vi "moveFilterWheel.vi"(6 "Delay between send and receive [ms]":i32=100, 8 "error in (no error)":errorcluster, 9 "position":i32, 10 "locationId":i32, 11 "Monochromator in":refnum<class "Monochromator.lvclass">) -> (0 "error out":errorcluster, 1 "ID":i32, 2 "results-JSON string":string, 3 "Monochromator out":refnum<class "Monochromator.lvclass">)   [LabVIEW 2023, in "Monochromator.lvclass"]
doc: "Move the filter wheel to a position.\n\nlocationId Integer. Specifies which filter wheel to move.\n0 = Filter wheel 1 (Internal)\n1 = Filter wheel 2 (External)\nposition Integer. Position to move the filter wheel."
uses:
  Monochromator.lvclass
  29a0d797-fd6c-43e0-b242-80b21aa51c30.vi
  7fe8abea-6ecd-46de-aa11-ce8637911b6a.vi
  35d46a5a-fd7c-4445-96f4-e877dae8f93b.vi
  <vilib>/JDP Science/JSONtext/Variant to JSON Text.vi
  <vilib>/JDP Science/JSONtext/Set Item.vi
  <vilib>/JDP Science/JSONtext/LVClass Serializer/JSONtext LVClass Serializer.lvclass
  Monochromator.lvclass/Monochromator.ctl
  GenericDevice/GenericDevice.lvclass
panel:
  # "Connector Pane"
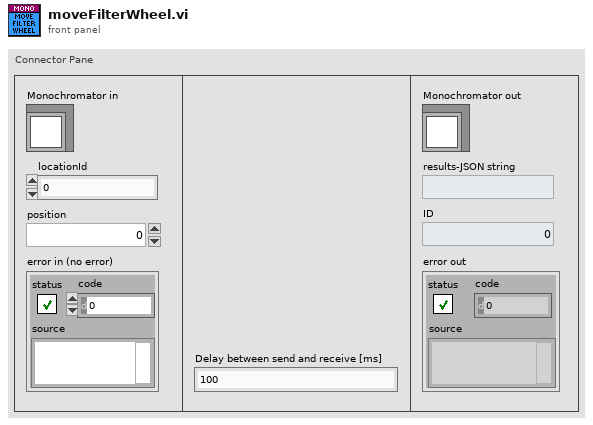
[diagram p1: front panel]
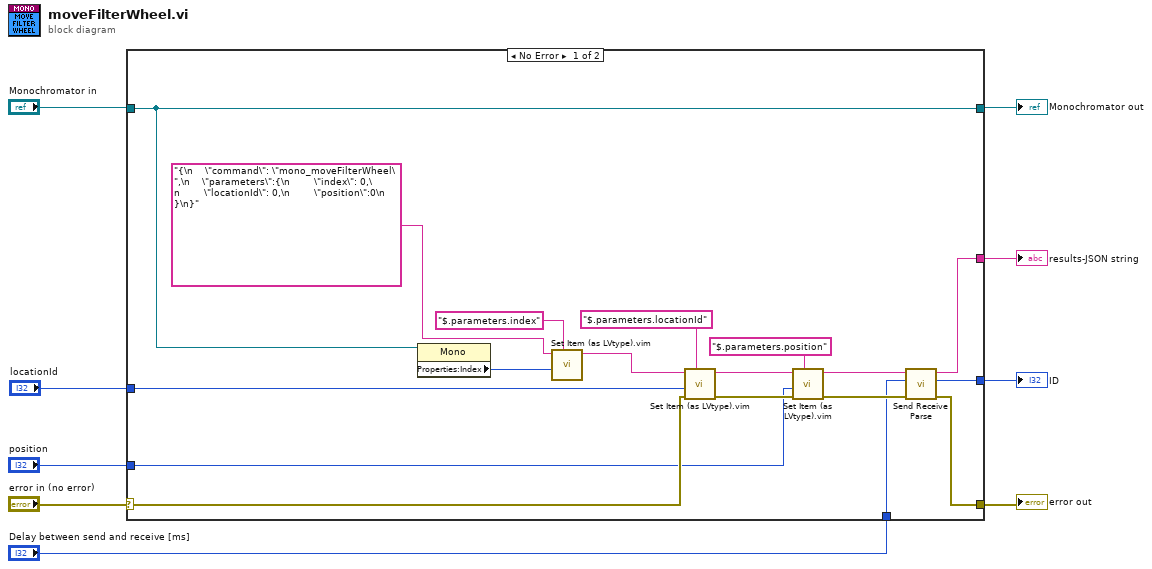
[diagram p0: block diagram]
diagram:
  n1 = case shown="No Error" "error in (no error)" {
    selector: "error in (no error)" -> [w26 w29]
    tunnel: [w23 w29] -> w6
    tunnel: [w15 w28] -> w8
    tunnel: "Monochromator in" -> [w15 w28]
    tunnel: [w25 _] -> w4
    tunnel: [w24 _] -> w5
    tunnel: "position" -> [w17 _]
    tunnel: "Delay between send and receive [ms]" -> [w16 _]
    tunnel: "locationId" -> [w10 _]
    frame No Error {
      n2 = property class="Mono"(reference=w15) -> ("Properties:Index"=w14:i32)  [unwired: 1 in, 2 out]
      n3 = call "Set Item (as LVtype).vim"("$Path or Item Name"="$.parameters.index", "Anything"=w14, "JSON"="{\n    \"command\": \"mono_moveFilterWheel\",\n    \"parameters\":{\n        \"index\": 0,\n        \"locationId\": 0,\n        \"position\":0\n    }\n}") -> ("<JSON>"=w12:string)  [unwired: 5 in, 2 out]
      n4 = call "Set Item (as LVtype).vim"("$Path or Item Name"="$.parameters.locationId", "error in (no error)"=w26, "Anything"=w10, "JSON"=w12) -> ("error out"=w21:errorcluster, "<JSON>"=w19:string)  [unwired: 4 in, 1 out]
      n5 = call "Set Item (as LVtype).vim"("$Path or Item Name"="$.parameters.position", "error in (no error)"=w21, "Anything"=w17, "JSON"=w19) -> ("error out"=w20:errorcluster, "<JSON>"=w18:string)  [unwired: 4 in, 1 out]
      n6 = call "Send Receive Parse.vi"("error in"=w20, "Delay between send and receive [ms]"=w16, "<JSON>"=w18) -> ("error out"=w23:errorcluster, "ID"=w24:i32, "results-JSON string"=w25:string)  [unwired: 6 in]
    }
    frame Error {
    }
  }
  "error out" <- w6
  "Monochromator out" <- w8
  "ID" <- w5
  "results-JSON string" <- w4
